vi "FTW-Actor-DynamicLaunchOptions.vi"() -> (0 "Open VI Ref Options":i32 format="%.0x")   [LabVIEW 2013, in "FTW-Actor.lvlib"]
uses:
  FTW-Actor.lvlib
panel:
  # "Inputs"
  # "Outputs"
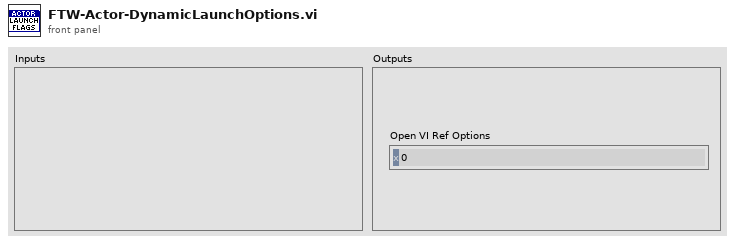
[diagram p1: front panel]
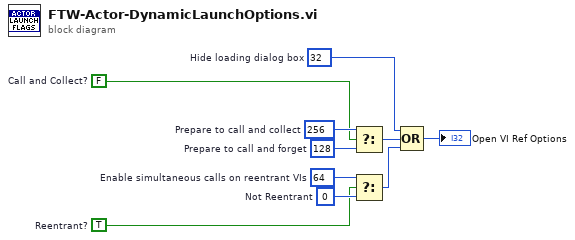
[diagram p0: block diagram]
diagram:
  w4 = TRUE  # Reentrant?
  w5 = FALSE  # Call and Collect?
  w1 = 32  # Hide loading dialog box
  w7 = 256  # Prepare to call and collect
  w8 = 0  # Not Reentrant
  w9 = 64  # Enable simultaneous calls on reentrant VIs
  w6 = 128  # Prepare to call and forget
  n1 = Select(t=w7, s=w5, f=w6) -> (s? t:f=w2:i32)
  n2 = Select(t=w9, s=w4, f=w8) -> (s? t:f=w3:i32)
  n3 = Compound Arithmetic op=OR(w1, w2, w3) -> (→"Open VI Ref Options":i32)
